vi "Car Control.vi"(7 "Reset":bool, 10 "Car Info":T2 {"Heading" format="%.1f"; "Y" format="%.3f"; "X" format="%.3f"; "Speed" format="%.2f"}, 11 "Ranges":T1 {"Rear" format="%.3f"; "Front" format="%.3f"}) -> (2 "Throttle (0 to 1)":sgl, 3 "Steering (-1 to 1)":sgl)   [LabVIEW 2020, in "Controller.lvlib"]
uses:
  Controller.lvlib
  FormulaG-Common/Car Info.ctl
  FormulaG-Common/Ranges.ctl
  FormulaG-Common/FormulaG-Common.lvlib
panel:
  out "Range Visualization":cluster{sgl[], sgl[]}[](graph)
  in  "Throttle":sgl(slide)=0.13636364 scale=0.0..1.0
  in  "Steering Sensitivity":sgl(slide)=0.6993007 scale=0.0..1.0
  # "Additional controls and indicators can be added to this VI to help with tuning control parameters and providing debugging info. This VI can be left open while the game runs so you can tweak its operation.\n\nEnsure you remember to set control value defaults by selecting them and choosing Make Selected Values Default in the Edit menu so parameters persist after closing the project, or you should change them to block diagram constants once they're set appropriately."
  # "** DO NOT CHANGE THE CONNECTOR PANE OF THIS VI **\nThese controls and indicators are for the standard inputs and outputs for this VI; trying to change these controls has no effect as they're set by the engine."
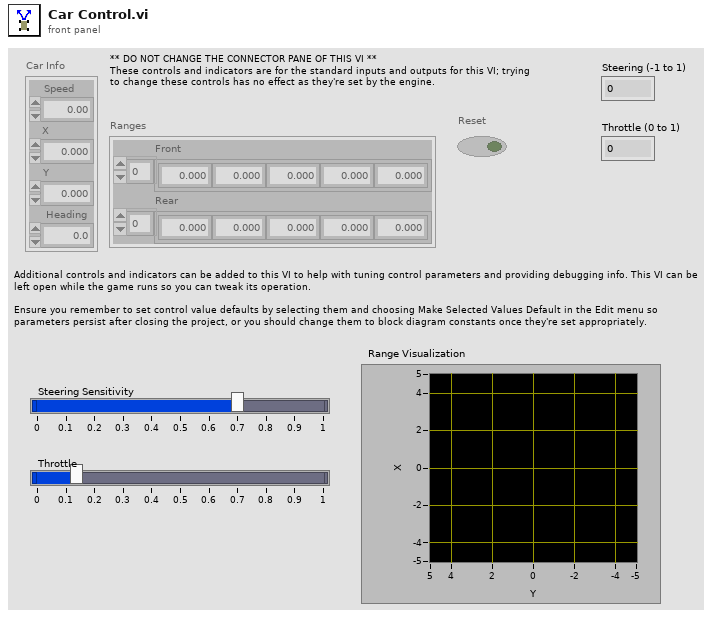
[diagram p1: front panel]
types:
  T1 = typedef "FormulaG-Common.lvlib/Ranges.ctl" = cluster{"Front":sgl[], "Rear":sgl[]}
  T2 = typedef "FormulaG-Common.lvlib/Car Info.ctl" = cluster{"Speed":sgl, "X":sgl, "Y":sgl, "Heading":sgl}
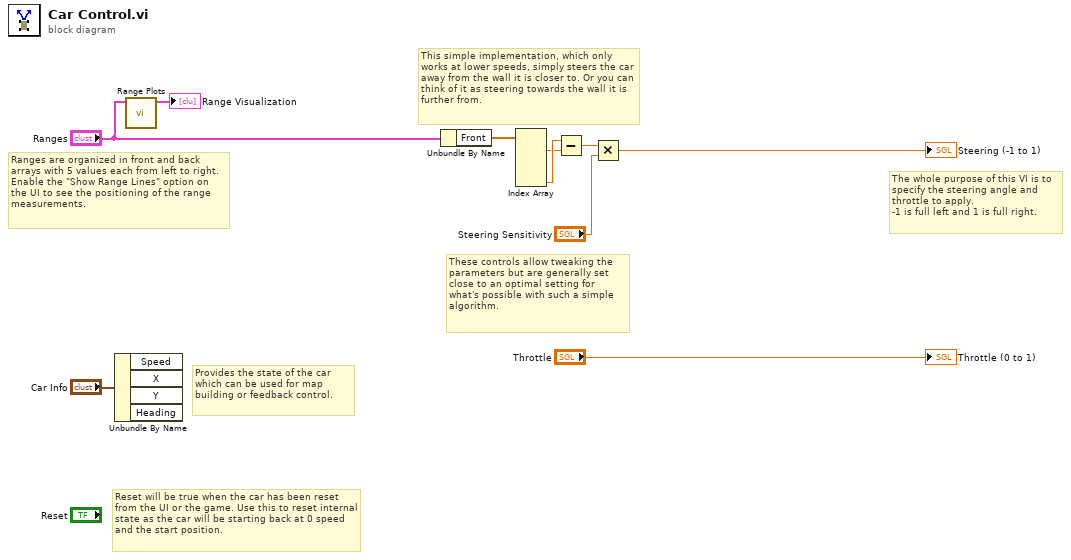
[diagram p0: block diagram]
diagram:
  # "The whole purpose of this VI is to specify the steering angle and throttle to apply.\n-1 is full left and 1 is full right."
  # "These controls allow tweaking the parameters but are generally set close to an optimal setting for what's possible with such a simple algorithm."
  # "This simple implementation, which only works at lower speeds, simply steers the car away from the wall it is closer to. Or you can think of it as steering towards the wall it is further from."
  # "Ranges are organized in front and back arrays with 5 values each from left to right. Enable the \"Show Range Lines\" option on the UI to see the positioning of the range measurements."
  # "Reset will be true when the car has been reset from the UI or the game. Use this to reset internal state as the car will be starting back at 0 speed and the start position."
  # "Provides the state of the car which can be used for map building or feedback control."
  n1 = Unbundle By Name("Car Info") -> ()  [unwired: 4 out]
  n2 = call "Range Plots.vi"("Ranges"="Ranges") -> ("Range Plots"=→"Range Visualization":cluster{sgl[], sgl[]}[])  [unwired: 10 in]
  n3 = Unbundle By Name("Ranges") -> ("Front"=w10:sgl[])
  n4 = Index Array(array=w10) -> (element #1=w8:sgl, element #5=w9:sgl)  [unwired: 5 in, 3 out]
  n5 = Subtract(x=w9, y=w8) -> (x-y=w7:sgl)
  n6 = Multiply(x=w7, y="Steering Sensitivity") -> (x*y=→"Steering (-1 to 1)":sgl)
  "Throttle (0 to 1)" <- "Throttle"
